vi "index state settings.vi"(3 "3-stop tubing":T4, 4 "Next Index":u32[](array[numeric]), 5 "State Settings":T1[][](array[typedef]) {"valve cycle time" min=0.2 step=0.1 format="%.2f"; "flow division"."5" min=0.0 max=1.0 step=0.01 format="%.3f"; "flow division"."4" min=0.0 max=1.0 step=0.01 format="%.3f"; "flow division"."3" min=0.0 max=1.0 step=0.01 format="%.3f"; "flow division"."2" min=0.0 max=1.0 step=0.01 format="%.3f"; "flow division"."1" min=0.0 max=1.0 step=0.01 format="%.3f"; "flow rate" format="%.3f"}) -> (0 "Controls":T5 {"Pump speed" format="%.2f"}, 1 "State":T1={"switches"={"Pump"=FALSE, "1"=FALSE, "2"=FALSE, "3"=FALSE, "4"=FALSE, "5"=FALSE, "6"=FALSE}, "flow rate"=0.0, "flow division"={"1"=0.0, "2"=0.0, "3"=0.0, "4"=0.0, "5"=0.0}, "State name"="", "state duration"=0.0, "valve cycle time"=0.2} {"valve cycle time" min=0.2 step=0.1 format="%.2f"; "flow division"."5" min=0.0 max=1.0 step=0.01 format="%.3f"; "flow division"."4" min=0.0 max=1.0 step=0.01 format="%.3f"; "flow division"."3" min=0.0 max=1.0 step=0.01 format="%.3f"; "flow division"."2" min=0.0 max=1.0 step=0.01 format="%.3f"; "flow division"."1" min=0.0 max=1.0 step=0.01 format="%.3f"; "flow rate" format="%.3f"})   [LabVIEW 2012]
uses:
  Peristaltic/pump rpm poly.vi/pump control.vi
  Stamp/Switch settings vertical.ctl
  flow fraction.ctl
  State Setting.ctl
  Stamp/Stamp Controls.ctl
  Peristaltic/3-stop colors.ctl
  switches.ctl
panel:
  # "rpm"
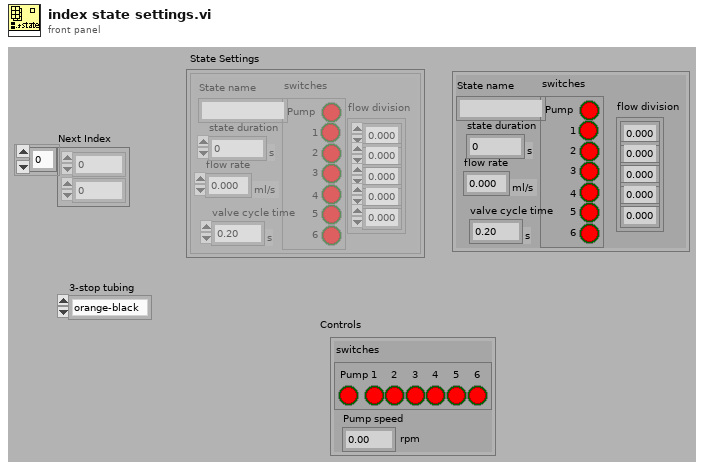
[diagram p1: front panel]
types:
  T1 = typedef "State Setting.ctl" = cluster{"switches":T2, "flow rate":dbl[unit], "flow division":cluster{"1":T3, "2":T3, "3":T3, "4":T3, "5":T3}, "State name":string, "state duration":dbl[unit], "valve cycle time":dbl[unit]}
  T2 = typedef "Switch settings vertical.ctl" = cluster{"Pump":bool, "1":bool, "2":bool, "3":bool, "4":bool, "5":bool, "6":bool}
  T3 = typedef "flow fraction.ctl" = dbl
  T4 = typedef "3-stop colors.ctl" = enum16{"orange-black", "orange-red", "orange-blue", "orange-green", "green-yellow", "orange-yellow", "white-yellow", "orange-white", "black-black", "orange-orange", "white-black", "white-white", "white-red", "red-red", "red-grey", "grey-grey", "yellow-yellow", "yellow-blue", "blue-blue", "blue-green", "green-green", "purple-purple", "purple-black", "purple-orange", "purple-white", "black-white", "13", "14", "15", "16", "17", "18"}
  T5 = typedef "Stamp Controls.ctl" = cluster{"Pump speed":dbl, "switches":T6}
  T6 = typedef "switches.ctl" = cluster{"Pump":bool, "1":bool, "2":bool, "3":bool, "4":bool, "5":bool, "6":bool}
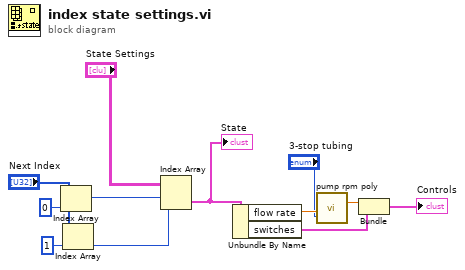
[diagram p0: block diagram]
diagram:
  n1 = Index Array(array="Next Index", index=0) -> (element=w11:u32)
  n2 = Index Array(array="Next Index", index=1) -> (element=w8:u32)
  n3 = Index Array(array="State Settings", index (row)=w11, index (col)=w8) -> (element=w1:T1)
  "State" <- w1
  n4 = Unbundle By Name(w1) -> ("flow rate"=w6:dbl[unit], "switches"=w3:T2)
  n5 = call-poly "pump rpm poly.vi"(0:w6, 1:"3-stop tubing") -> ("pump speed (rpm)"=w4:dbl)  [unwired: 2 in, 1 out]
  n6 = Bundle("pump speed (rpm)"=w4, "switches"=w3) -> (→"Controls":cluster{"pump speed (rpm)":dbl, "switches":T2})  [unwired: 1 in]
